vi "Set Result Settings.vi"(8 "error in (no error)":errorcluster, 10 "Analyze Results":refnum<class "Analyze Results Base.lvclass">, 11 "Analyze BaseClass in":refnum<class "HIJ Vision Application.lvclass">) -> (0 "error out":errorcluster, 3 "Analyze BaseClass out":refnum<class "HIJ Vision Application.lvclass">)   [LabVIEW 2020, in "HIJ Vision Application.lvlib" / "HIJ Vision Application.lvclass"]
uses:
  HIJ Vision Application.lvclass
  Analyze/Results and Overlays/Results Base/Analyze Results Base.lvclass
  HIJ Vision Application.lvclass/HIJ Vision Application.ctl
  Analyze/Analyze Actor/Analyze Actor Messages/Set Result Settings Msg/Set Result Settings Msg.lvclass
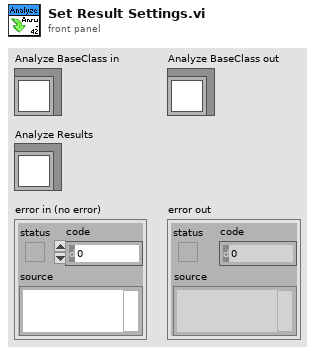
[diagram p1: front panel]
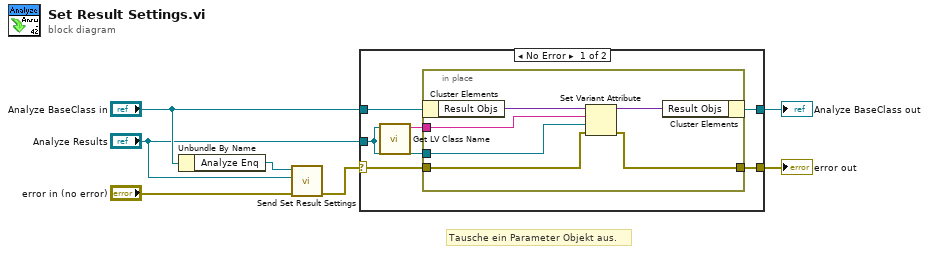
[diagram p0: block diagram]
diagram:
  # "Tausche ein Parameter Objekt aus."
  n1 = Unbundle By Name("Analyze BaseClass in") -> ("Analyze Enq"=w3:refnum<class "Message Enqueuer.lvclass">)
  n2 = call "Send Set Result Settings.vi"("error in (no error)"="error in (no error)", "Analyze Parameter"="Analyze Results", "Message Enqueuer"=w3) -> ("error out"=w1:errorcluster)  [unwired: 7 in, 1 out]
  n3 = case shown="No Error" w1 {
    selector: w1 -> [w10 w21]
    tunnel: [w9 w21] -> w7
    tunnel: [w8 w20] -> w6
    tunnel: "Analyze BaseClass in" -> [w13 w20]
    tunnel: "Analyze Results" -> [w11 _]
    frame No Error {
      n4 = call <vilib>:"Get LV Class Name.vi"("object"=w11) -> ("class name"=w12:string)  [unwired: 9 in, 1 out]
      n5 = in-place {
        in-place-border: w12 -> [w19]
        in-place-border: w11 -> [w18]
        in-place-border: w10 -> [w15]
        in-place-border: [w14] -> w9
        n6 = in-place-cluster #1(w13) -> ("Result Objs"=w17:variant)
        n7 = Set Variant Attribute(Variant=w17, name=w19, value=w18, error in=w15) -> (Variant out=w16:variant, error out=w14:errorcluster)  [unwired: 1 out]
        n8 = in-place-cluster #1("Result Objs"=w16) -> (w8:refnum<class "HIJ Vision Application.lvclass">)
      }
    }
    frame Error {
    }
  }
  "error out" <- w7
  "Analyze BaseClass out" <- w6
